vi "focusKnobOpen.vi"   [LabVIEW 2017]
uses:
  globalDevices.vi
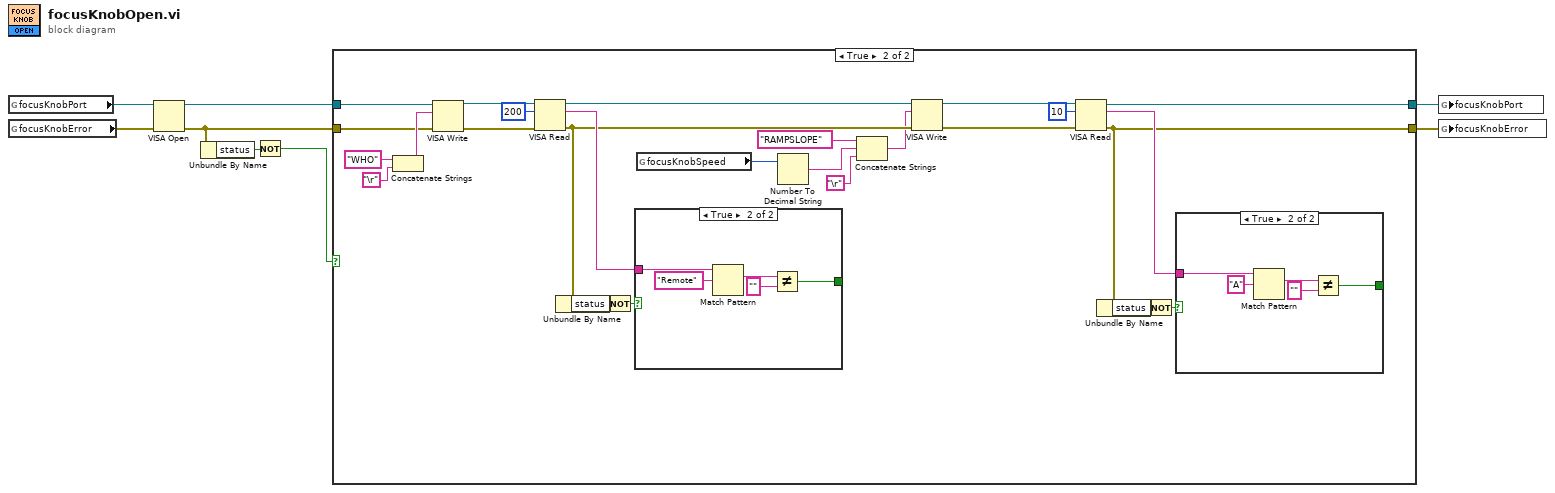
[diagram p0: block diagram]
diagram:
  n1 = global read "globalDevices.vi" "focusKnobPort"() -> (w8:refnum<visa-resource-name>)
  n2 = global read "globalDevices.vi" "focusKnobError"() -> (w7:errorcluster)
  n3 = VISA Open(error in (no error)=w7, VISA resource name=w8) -> (VISA resource name=w6:refnum<visa-resource-name>, error out=w3:errorcluster)  [unwired: 3 in]
  n4 = Unbundle By Name(w3) -> ("status"=w2:bool)
  n5 = Not(x=w2) -> (.not. x?=w1:bool)
  n6 = case shown="True" w1 {
    tunnel: w6 -> [w10 w36]
    tunnel: [w10 w13] -> w5
    tunnel: [w9 w12] -> w4
    tunnel: w3 -> [w9 w11]
    frame False {
    }
    frame True {
      n7 = Concatenate Strings("WHO" ("write buffer"), "\r") -> (w35:string)
      n8 = VISA Write(VISA resource name=w36, write buffer=w35, error in (no error)=w11) -> (VISA resource name out=w32:refnum<visa-resource-name>, error out=w30:errorcluster)  [unwired: 1 out]
      n9 = VISA Read(VISA resource name=w32, byte count=u32 200, error in (no error)=w30) -> (VISA resource name out=w26:refnum<visa-resource-name>, read buffer=w28:string, error out=w25:errorcluster)  [unwired: 1 out]
      n10 = Unbundle By Name(w25) -> ("status"=w29:bool)
      n11 = Not(x=w29) -> (.not. x?=w27:bool)
      n12 = case shown="True" w27 {
        selector: w27 -> [w43 _]
        tunnel: w28 -> [_ w48]
        tunnel: [w43 w44] -> _
        frame False {
        }
        frame True {
          n13 = Match Pattern(string=w48, regular expression="Remote") -> (match substring=w46:string)  [unwired: 1 in, 3 out]
          n14 = Not Equal?(x=w46, y="") -> (x != y?=w44:bool)
        }
      }
      n15 = global read "globalDevices.vi" "focusKnobSpeed"() -> (w21:u8)
      n16 = Number To Decimal String(number=w21) -> (decimal integer string=w22:string)  [unwired: 1 in]
      n17 = Concatenate Strings("RAMPSLOPE" ("write buffer"), w22, "\r") -> (w20:string)
      n18 = VISA Write(VISA resource name=w26, write buffer=w20, error in (no error)=w25) -> (VISA resource name out=w19:refnum<visa-resource-name>, error out=w18:errorcluster)  [unwired: 1 out]
      n19 = VISA Read(VISA resource name=w19, byte count=u32 10, error in (no error)=w18) -> (VISA resource name out=w13:refnum<visa-resource-name>, read buffer=w14:string, error out=w12:errorcluster)  [unwired: 1 out]
      n20 = Unbundle By Name(w12) -> ("status"=w15:bool)
      n21 = Not(x=w15) -> (.not. x?=w16:bool)
      n22 = case shown="True" w16 {
        selector: w16 -> [w37 _]
        tunnel: w14 -> [_ w42]
        tunnel: [w37 w38] -> _
        frame False {
        }
        frame True {
          n23 = Match Pattern(string=w42, regular expression="A") -> (match substring=w40:string)  [unwired: 1 in, 3 out]
          n24 = Not Equal?(x=w40, y="") -> (x != y?=w38:bool)
        }
      }
    }
  }
  n25 = global write "globalDevices.vi" "focusKnobPort"(w5) -> ()
  n26 = global write "globalDevices.vi" "focusKnobError"(w4) -> ()
